vi "row2.vi"(2 "Array in":i32[](array[numeric])) -> (0 "Array out":i32[](array[numeric]), 1 "Enum":T1(ring))   [LabVIEW 2016]
uses:
  <vilib>/NXT/Block Support/NXT_OutputPort.ctl
  <vilib>/NXT/Block Support/NXT_InputPort.ctl
  <vilib>/NXT/Subs/ColorSensorColors.ctl
  <vilib>/NXT/NXTIO Xnodes/NXTIONodeSubVIs/NXTStopMotors.vi
  <vilib>/NXT/NXTIO Xnodes/NXTIONodeSubVIs/NXTMotorRunDistance.vi
  <vilib>/NXT/NXTIO Xnodes/NXTIONodeSubVIs/LEGOMotorStatus.vi
  <vilib>/NXT/NXTIO Xnodes/NXTIONodeSubVIs/NXTMoveMotors.vi
  <vilib>/NXT/NXTIO Xnodes/NXTIONodeSubVIs/LEGOResetMotors.vi
  <vilib>/NXT/Subs/LVHSConnector.ctl
  <vilib>/NXT/NXTIO Xnodes/AddressXNode/NXTIOAddress.xnode
  <vilib>/NXT/NXTIO Xnodes/NXTIOXNode/NXTIO.xnode
  <vilib>/NXT/LegoClasses/BrickReference/BrickReference.lvclass
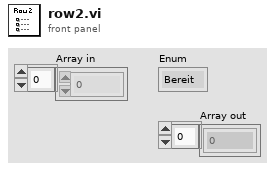
[diagram p1: front panel]
types:
  T1 = enum16{"Bereit", "Move 1", "Reference_pos", "Wait", "row1_check", "row2_check", "row3_check", "return", "move2", "move3", "move4", "move5", "end"}
  T2 = enum16{"forward", "pause1", "left1", "pause2", "left2", "pause3", "end"}
  T3 = typedef "NXT_OutputPort.ctl" = u8
  T4 = typedef "ColorSensorColors.ctl" = enum16{"No Color", "Black", "Blue", "Green", "Yellow", "Red", "White", "Brown"}
  T5 = cluster{"Output Port":T3, "Output Port 2":T3, "Output Port 3":T3}
  T6 = typedef "LVHSConnector.ctl" = refnum<class "BrickReference.lvclass">
  T7 = typedef "NXT_InputPort.ctl" = u32
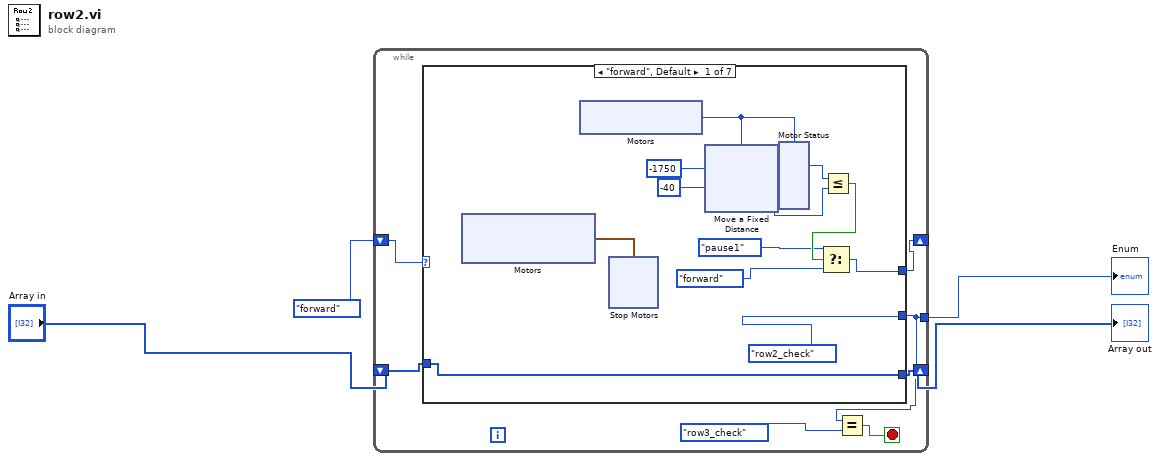
[diagram p0: block diagram]
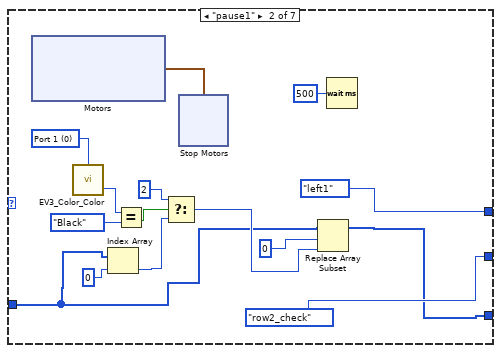
[diagram p2: hidden frame]
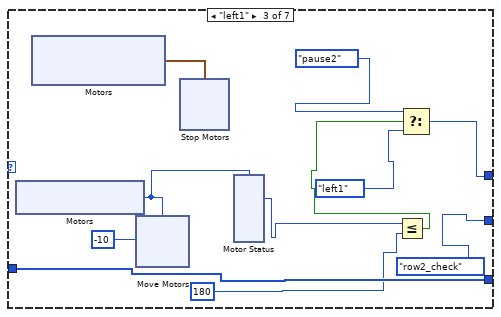
[diagram p3: hidden frame]
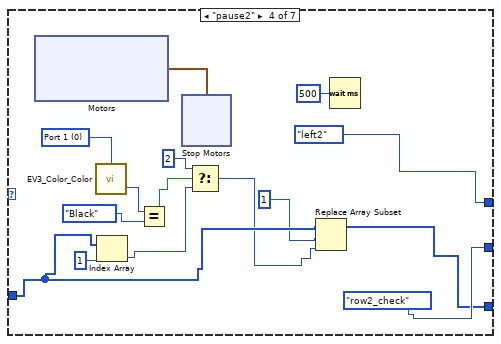
[diagram p4: hidden frame]
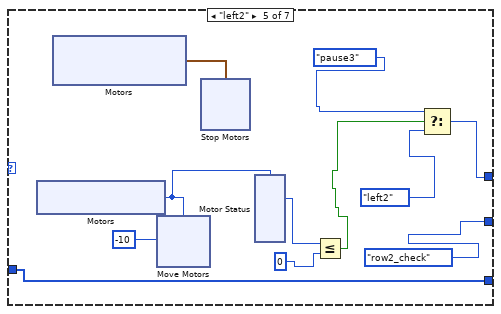
[diagram p5: hidden frame]
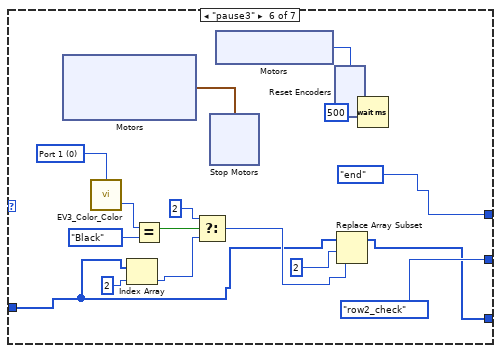
[diagram p6: hidden frame]
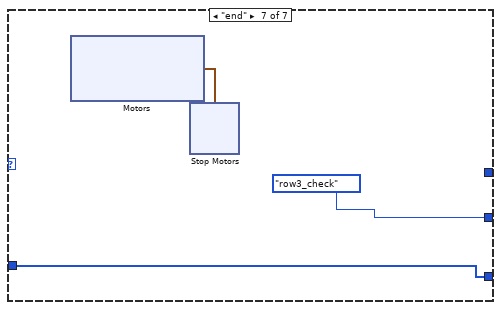
[diagram p7: hidden frame]
diagram:
  n1 = while {
    shift-right: [w6] -> _
    shift-left: T2."forward" -> [w7]
    tunnel: [w10] -> w3
    shift-right: [w8] -> w2
    shift-left: "Array in" -> [w9]
    stop <- w11 stop-if-true
    n2 = case shown="\"forward\", Default" w7 {
      tunnel: [w12 T2."left1" w77 T2."left2" w131 T2."end" _] -> w6
      tunnel: [T1."row2_check" T1."row2_check" T1."row2_check" T1."row2_check" T1."row2_check" T1."row2_check" T1."row3_check"] -> w10
      tunnel: [w22 w52 w76 w103 w130 w163 w185] -> w8
      tunnel: w9 -> [w22 w50 w76 w106 w130 w159 w185]
      frame "forward", Default {
        w18 = -1750 ("Distance 1")
        n3 = xnode "Motors"() -> ("Motor"=w23:cluster{"Port":T3, "Port":T3})
        n4 = xnode "Motors"() -> ("Motor"=w17:T3)
        n5 = xnode "Stop Motors"("Motors"=w23) -> ()  [unwired: 1 in, 1 out]
        n6 = xnode "Move a Fixed Distance"("Speed 1"=i8 -40, "Distance 1"=w18, "Motors"=w17) -> ("NXT/EV3"=w16:T6)  [unwired: 1 in]
        n7 = xnode "Motor Status"("Motors"=w17, "NXT/EV3"=w16) -> ("Position 1"=w19:i32)  [unwired: 2 out]
        n8 = Less Or Equal?(x=w19, y=w18) -> (x <= y?=w15:bool)
        n9 = Select(t=T2."pause1", s=w15, f=T2."forward") -> (s? t:f=w12:T2)
      }
      frame "pause1" {
        w62 = T7 0 items=["Port 1", "Port 2", "Port 3", "Port 4"] ("Port (Port 1)")
        n10 = xnode "Motors"() -> ("Motor"=w63:cluster{"Port":T3, "Port":T3, "Port":T3})
        n11 = call <vilib>:"EV3_Color_Color.vi"("Port (Port 1)"=w62) -> ("Detected Color"=w61:T4)  [unwired: 2 in, 1 out]
        n12 = Index Array(array=w50, index=0 ("disabled index (col)")) -> (element=w49:i32)
        n13 = Equal?(x=w61, y=ColorSensorColors."Black") -> (x = y?=w58:bool)
        n14 = Select(t=2 ("disabled index (col)"), s=w58, f=w49) -> (s? t:f=w53:i32)
        n15 = xnode "Stop Motors"("Motors"=w63) -> ()  [unwired: 1 in, 1 out]
        n16 = Replace Array Subset(array=w50, new element=w53, index=0 ("disabled index (col)")) -> (w52:i32[])
        n17 = Wait (ms)(milliseconds to wait=u32 500) -> ()  [unwired: 1 out]
      }
      frame "left1" {
        n18 = xnode "Motors"() -> ("Motor"=w79:T3)
        n19 = xnode "Motors"() -> ("Motor"=w78:cluster{"Port":T3, "Port":T3})
        n20 = xnode "Move Motors"("Power/Speed 1"=i8 -10, "Motors"=w79) -> ()  [unwired: 1 in, 1 out]
        n21 = xnode "Stop Motors"("Motors"=w78) -> ()  [unwired: 1 in, 1 out]
        n22 = xnode "Motor Status"("Motors"=w79) -> ("Position 1"=w73:i32)  [unwired: 1 in, 2 out]
        n23 = Less Or Equal?(x=w73, y=180) -> (x <= y?=w71:bool)
        n24 = Select(t=T2."pause2", s=w71, f=T2."left1") -> (s? t:f=w77:T2)
      }
      frame "pause2" {
        w116 = T7 0 items=["Port 1", "Port 2", "Port 3", "Port 4"] ("Port (Port 1)")
        n25 = xnode "Motors"() -> ("Motor"=w117:cluster{"Port":T3, "Port":T3, "Port":T3})
        n26 = call <vilib>:"EV3_Color_Color.vi"("Port (Port 1)"=w116) -> ("Detected Color"=w115:T4)  [unwired: 2 in, 1 out]
        n27 = Index Array(array=w106, index=1 ("disabled index (col)")) -> (element=w107:i32)
        n28 = Equal?(x=w115, y=ColorSensorColors."Black") -> (x = y?=w112:bool)
        n29 = xnode "Stop Motors"("Motors"=w117) -> ()  [unwired: 1 in, 1 out]
        n30 = Select(t=2 ("disabled index (col)"), s=w112, f=w107) -> (s? t:f=w104:i32)
        n31 = Replace Array Subset(array=w106, new element=w104, index=1 ("index (row)")) -> (w103:i32[])
        n32 = Wait (ms)(milliseconds to wait=u32 500) -> ()  [unwired: 1 out]
      }
      frame "left2" {
        n33 = xnode "Motors"() -> ("Motor"=w133:T3)
        n34 = xnode "Motors"() -> ("Motor"=w132:cluster{"Port":T3, "Port":T3})
        n35 = xnode "Move Motors"("Power/Speed 1"=i8 -10, "Motors"=w133) -> ()  [unwired: 1 in, 1 out]
        n36 = xnode "Stop Motors"("Motors"=w132) -> ()  [unwired: 1 in, 1 out]
        n37 = xnode "Motor Status"("Motors"=w133) -> ("Position 1"=w129:i32)  [unwired: 1 in, 2 out]
        n38 = Less Or Equal?(x=w129, y=0) -> (x <= y?=w127:bool)
        n39 = Select(t=T2."pause3", s=w127, f=T2."left2") -> (s? t:f=w131:T2)
      }
      frame "pause3" {
        w171 = T7 0 items=["Port 1", "Port 2", "Port 3", "Port 4"] ("Port (Port 1)")
        n40 = xnode "Motors"() -> ("Motor"=w172:cluster{"Port":T3, "Port":T3, "Port":T3})
        n41 = call <vilib>:"EV3_Color_Color.vi"("Port (Port 1)"=w171) -> ("Detected Color"=w170:T4)  [unwired: 2 in, 1 out]
        n42 = Index Array(array=w159, index=2 ("disabled index (col)")) -> (element=w158:i32)
        n43 = Equal?(x=w170, y=ColorSensorColors."Black") -> (x = y?=w167:bool)
        n44 = Select(t=2 ("disabled index (col)"), s=w167, f=w158) -> (s? t:f=w161:i32)
        n45 = xnode "Stop Motors"("Motors"=w172) -> ()  [unwired: 1 in, 1 out]
        n46 = xnode "Motors"() -> ("Motor"=w157:T3)
        n47 = xnode "Reset Encoders"("Motors"=w157) -> ()  [unwired: 1 in, 1 out]
        n48 = Replace Array Subset(array=w159, new element=w161, index=2 ("disabled index (col)")) -> (w163:i32[])
        n49 = Wait (ms)(milliseconds to wait=u32 500) -> ()  [unwired: 1 out]
      }
      frame "end" {
        n50 = xnode "Motors"() -> ("Motor"=w186:cluster{"Port":T3, "Port":T3, "Port":T3})
        n51 = xnode "Stop Motors"("Motors"=w186) -> ()  [unwired: 1 in, 1 out]
      }
    }
    n52 = Equal?(x=w10, y=T1."row3_check") -> (x = y?=w11:bool)
  }
  "Enum" <- w3
  "Array out" <- w2
